vi "Brent Search Powell.vi"(1 "p":dbl[](array[numeric]) format="%.2f", 2 "xit":dbl[](array[numeric]) format="%.2f", 3 "ZEPS":dbl=1e-12 format="%.2e", 6 "Parsed Formula":cluster{"table":i32[][], "result":dbl[]}, 7 "Variables":i32[](array[numeric])=[0, 0], 8 "tol":dbl=1e-06 format="%.2e", 9 "c (start)":dbl=1.0 format="%.2f", 10 "b (start)":dbl=0.5 format="%.2f", 11 "a (start)":dbl format="%.2f") -> (0 "u":dbl=1.5920119327128747e-12 format="%.2f")   [LabVIEW 2024, in "NI_Gmath.lvlib"]
uses:
  NI_Gmath.lvlib
panel:
  in  "fx":dbl=3.25 format="%.2f"
  in  "fw":dbl=2.000000000005184 format="%.2f"
  in  "fv":dbl=2.000000000008388 format="%.2f"
  in  "fu":dbl=2.000000000003184 format="%.2f"
  in  "e":dbl format="%.2f"
  in  "b":dbl format="%.2f"
  in  "a":dbl format="%.2f"
  in  "x":dbl=0.5 format="%.2f"
  in  "w":dbl=2.5920145247273993e-12 format="%.2f"
  in  "v":dbl=4.1939676003423364e-12 format="%.2f"
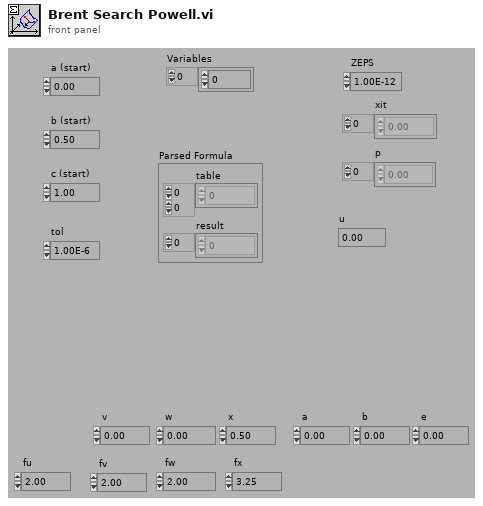
[diagram p1: front panel]
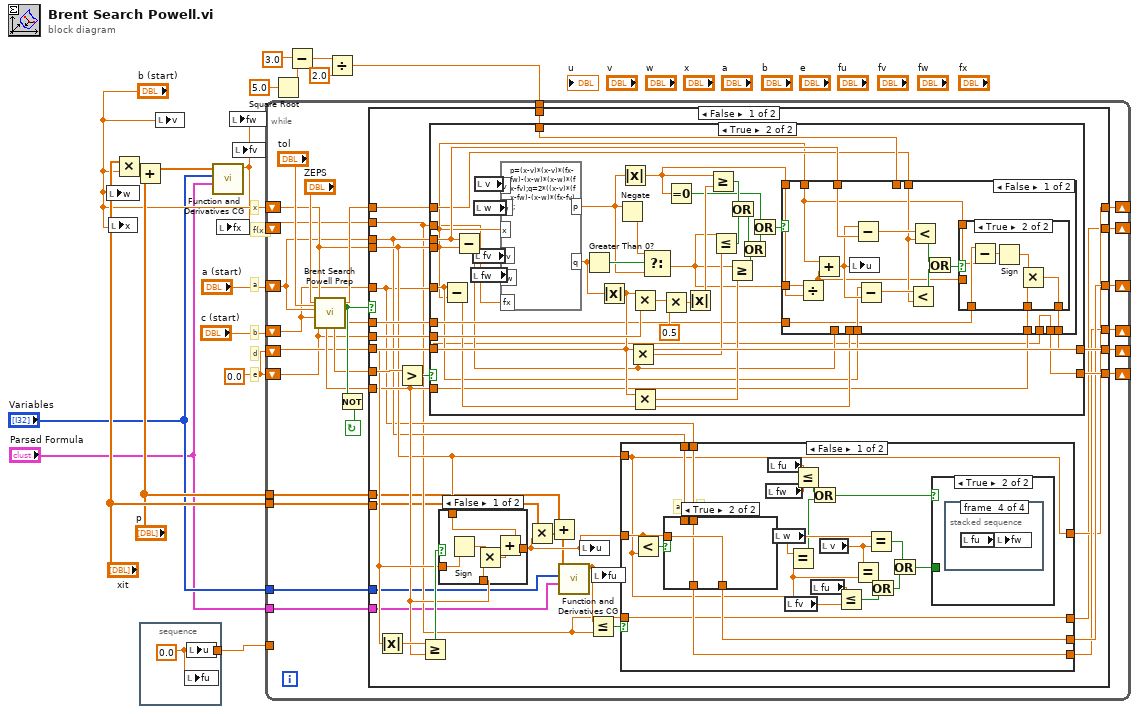
[diagram p0: block diagram]
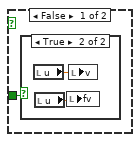
[diagram p2: hidden frame]
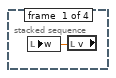
[diagram p4: hidden frame]
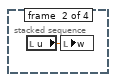
[diagram p5: hidden frame]
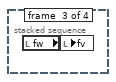
[diagram p6: hidden frame]
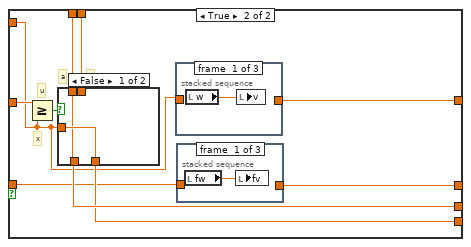
[diagram p8: hidden frame]
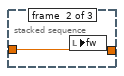
[diagram p9: hidden frame]
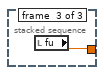
[diagram p10: hidden frame]
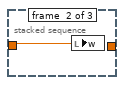
[diagram p11: hidden frame]
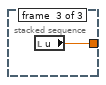
[diagram p12: hidden frame]
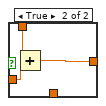
[diagram p14: hidden frame]
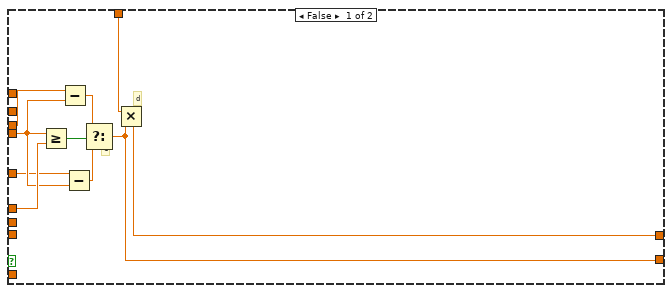
[diagram p15: hidden frame]
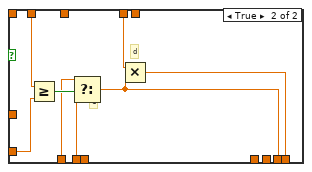
[diagram p17: hidden frame]
diagram:
  w11 = 0.0
  # "d"
  # "e"
  # "f(x)"
  # "x"
  # "b"
  # "a"
  n1 = local write "w"("b (start)") -> ()
  n2 = local write "x"("b (start)") -> ()
  n3 = Multiply(x="xit", y="b (start)") -> (x*y=w10:dbl[])
  n4 = Add(x=w10, y="p") -> (x+y=w9:dbl[])
  n5 = stacked-sequence {
    tunnel: [w19] -> w3
    frame #0 {
      w19 = 0.0
      n6 = local write "fu"(w19) -> ()
      n7 = local write "u"(w19) -> ()
    }
  }
  n8 = local write "v"("b (start)") -> ()
  n9 = call "Function and Derivatives CG.vi"("Parsed Formula"="Parsed Formula", "Variables"="Variables", "X"=w9) -> ("f(X)"=w4:dbl)  [unwired: 7 in, 1 out]
  n10 = local write "fx"(w4) -> ()
  n11 = local write "fw"(w4) -> ()
  n12 = local write "fv"(w4) -> ()
  n13 = Square Root(x=5.0) -> (sqrt(x)=w16:dbl)
  n14 = Subtract(x=3.0, y=w16) -> (x-y=w15:dbl)
  n15 = Divide(x=w15, y=2.0) -> (x/y=w12:dbl)
  n16 = while {
    tunnel: w3 -> [_]
    tunnel: "p" -> [w23]
    tunnel: "xit" -> [w22]
    shift-left: w11 -> [w29]
    shift-right: [w30] -> _
    tunnel: w12 -> [w32]
    shift-left: w11 -> [w28]
    shift-right: [w31] -> _
    shift-left: w4 -> [w36]
    shift-right: [w24] -> _
    shift-left: "b (start)" -> [w41]
    shift-right: [w25] -> _
    shift-left: "c (start)" -> [w33]
    shift-right: [w26] -> _
    shift-left: "a (start)" -> [w34]
    shift-right: [w27] -> _
    tunnel: "Variables" -> [w21]
    tunnel: "Parsed Formula" -> [w20]
    stop <- w39 continue-if-true
    n17 = call "Brent Search Powell Prep.vi"("ZEPS"="ZEPS", "e"=w28, "c (start)"=w33, "tol"="tol", "a (start)"=w34, "b (start)"=w41) -> ("value a"=w35:dbl, "value b"=w38:dbl, "convergence?"=w40:bool, "tol2"=w42:dbl, "value c"=w37:dbl)
    n18 = Not(x=w40) -> (.not. x?=w39:bool)
    n19 = case shown="False" w40 {
      tunnel: w41 -> [w59 _]
      tunnel: w38 -> [w73 w220]
      tunnel: w37 -> [w62 _]
      tunnel: w36 -> [w52 w218]
      tunnel: w35 -> [w71 _]
      tunnel: w34 -> [w58 w217]
      tunnel: w33 -> [w57 w216]
      tunnel: w32 -> [w70 _]
      tunnel: [w69 w220] -> w31
      tunnel: [w63 w221] -> w30
      tunnel: w29 -> [w68 w221]
      tunnel: w28 -> [w67 _]
      tunnel: w42 -> [w66 w219]
      tunnel: [w56 w217] -> w27
      tunnel: [w55 w216] -> w26
      tunnel: [w54 w219] -> w25
      tunnel: [w53 w218] -> w24
      tunnel: w22 -> [w50 _]
      tunnel: w23 -> [w47 _]
      tunnel: w21 -> [w46 _]
      tunnel: w20 -> [w45 _]
      frame False {
        n20 = Greater?(x=w73, y=w62) -> (0:w72:bool)
        n21 = case shown="True" w72 {
          tunnel: w59 -> [w141 w152]
          tunnel: w52 -> [_ w151]
          tunnel: w71 -> [w145 w164]
          tunnel: w58 -> [w140 w157]
          tunnel: w57 -> [w139 w156]
          tunnel: w70 -> [w138 w161]
          tunnel: [w137 w159] -> w69
          tunnel: [w136 w160] -> w63
          tunnel: w68 -> [_ w153]
          tunnel: w67 -> [_ w177]
          tunnel: w66 -> [_ w155]
          tunnel: w62 -> [_ w154]
          frame False {
            # "d"
            # "e"
            n22 = Greater Or Equal?(x=w141, y=w145) -> (x >= y?=w144:bool)
            n23 = Subtract(x=w140, y=w141) -> (x-y=w142:dbl)
            n24 = Subtract(x=w139, y=w141) -> (x-y=w143:dbl)
            n25 = Select(t=w142, s=w144, f=w143) -> (s? t:f=w137:dbl)
            n26 = Multiply(x=w138, y=w137) -> (x*y=w136:dbl)
          }
          frame True {
            n27 = Subtract(x=w156, y=w152) -> (x-y=w162:dbl)
            n28 = Subtract(x=w157, y=w152) -> (x-y=w163:dbl)
            n29 = local read "fw"() -> (w180:dbl)
            n30 = local read "fv"() -> (w181:dbl)
            n31 = local read "w"() -> (w182:dbl)
            n32 = local read "v"() -> (w183:dbl)
            n33 = formula code="p=(x-v)*(x-v)*(fx-fw)-(x-w)*(x-w)*(fx-fv);q=2*((x-v)*(fx-fw)-(x-w)*(fx-fv));"("v"=w183, "w"=w182, "x"=w152, "fv"=w181, "fw"=w180, "fx"=w151) -> ("p"=w147:dbl, "q"=w172:dbl)
            n34 = Greater Than 0?(x=w172) -> (x > 0?=w179:bool)
            n35 = Absolute Value(x=w172) -> (abs(x)=w171:dbl)
            n36 = Negate(x=w147) -> (-x=w178:dbl)
            n37 = Absolute Value(x=w147) -> (abs(x)=w146:dbl)
            n38 = Multiply(x=w171, y=w163) -> (x*y=w170:dbl)
            n39 = Multiply(x=w171, y=w177) -> (x*y=w176:dbl)
            n40 = Multiply(x=w171, y=w162) -> (x*y=w169:dbl)
            n41 = Select(t=w178, s=w179, f=w147) -> (s? t:f=w158:dbl)
            n42 = Multiply(x=w176, y=0.5) -> (x*y=w174:dbl)
            n43 = Equal To 0?(x=w146) -> (x = 0?=w149:bool)
            n44 = Absolute Value(x=w174) -> (abs(x)=w173:dbl)
            n45 = Greater Or Equal?(x=w146, y=w173) -> (x >= y?=w168:bool)
            n46 = Less Or Equal?(x=w158, y=w170) -> (x <= y?=w167:bool)
            n47 = Greater Or Equal?(x=w158, y=w169) -> (x >= y?=w165:bool)
            n48 = Or(x=w168, y=w167) -> (x .or. y?=w166:bool)
            n49 = Or(x=w166, y=w165) -> (x .or. y?=w150:bool)
            n50 = Or(x=w149, y=w150) -> (x .or. y?=w148:bool)
            n51 = case shown="False" w148 {
              tunnel: w152 -> [w187 w214]
              tunnel: w164 -> [w188 w213]
              tunnel: w163 -> [_ w212]
              tunnel: w162 -> [_ w211]
              tunnel: w161 -> [_ w210]
              tunnel: [w185 w209] -> w160
              tunnel: [w184 w208] -> w159
              tunnel: w158 -> [w200 _]
              tunnel: w146 -> [w199 _]
              tunnel: w157 -> [w198 _]
              tunnel: w156 -> [w196 _]
              tunnel: w155 -> [w193 _]
              tunnel: w154 -> [w186 _]
              tunnel: w153 -> [w184 _]
              frame False {
                n52 = Divide(x=w200, y=w199) -> (x/y=w189:dbl)
                n53 = Add(x=w187, y=w189) -> (x+y=w197:dbl)
                n54 = local write "u"(w197) -> ()
                n55 = Subtract(x=w197, y=w198) -> (x-y=w195:dbl)
                n56 = Subtract(x=w196, y=w197) -> (x-y=w194:dbl)
                n57 = Less?(x=w194, y=w193) -> (x < y?=w191:bool)
                n58 = Less?(x=w195, y=w193) -> (x < y?=w192:bool)
                n59 = Or(x=w192, y=w191) -> (x .or. y?=w190:bool)
                n60 = case shown="True" w190 {
                  tunnel: w189 -> [w201 _]
                  tunnel: w188 -> [_ w207]
                  tunnel: w187 -> [_ w206]
                  tunnel: w186 -> [_ w203]
                  tunnel: [w201 w202] -> w185
                  frame False {
                  }
                  frame True {
                    n61 = Subtract(x=w207, y=w206) -> (x-y=w205:dbl)
                    n62 = Sign(1:w205) -> (0:w204:dbl)
                    n63 = Multiply(x=w204, y=w203) -> (x*y=w202:dbl)
                  }
                }
              }
              frame True {
                # "d"
                # "e"
                n64 = Greater Or Equal?(x=w214, y=w213) -> (x >= y?=w215:bool)
                n65 = Select(t=w212, s=w215, f=w211) -> (s? t:f=w208:dbl)
                n66 = Multiply(x=w210, y=w208) -> (x*y=w209:dbl)
              }
            }
          }
        }
        n67 = Absolute Value(x=w63) -> (abs(x)=w64:dbl)
        n68 = Greater Or Equal?(x=w64, y=w62) -> (x >= y?=w65:bool)
        n69 = case shown="False" w65 {
          tunnel: w63 -> [w132 w135]
          tunnel: w59 -> [w128 w134]
          tunnel: w62 -> [w130 _]
          tunnel: [w127 w133] -> w51
          frame False {
            n70 = Sign(1:w132) -> (0:w131:dbl)
            n71 = Multiply(x=w131, y=w130) -> (x*y=w129:dbl)
            n72 = Add(x=w128, y=w129) -> (x+y=w127:dbl)
          }
          frame True {
            n73 = Add(x=w134, y=w135) -> (x+y=w133:dbl)
          }
        }
        n74 = Multiply(x=w50, y=w51) -> (x*y=w49:dbl[])
        n75 = Add(x=w47, y=w49) -> (x+y=w48:dbl[])
        n76 = call "Function and Derivatives CG.vi"("Parsed Formula"=w45, "Variables"=w46, "X"=w48) -> ("f(X)"=w61:dbl)  [unwired: 7 in, 1 out]
        n77 = local write "u"(w51) -> ()
        n78 = Less Or Equal?(x=w61, y=w52) -> (x <= y?=w60:bool)
        n79 = local write "fu"(w61) -> ()
        n80 = case shown="False" w60 {
          tunnel: w51 -> [w92 w116]
          tunnel: w59 -> [w75 w110]
          tunnel: w58 -> [w94 w114]
          tunnel: w57 -> [w93 w113]
          tunnel: [w90 w112] -> w56
          tunnel: [w91 w111] -> w55
          tunnel: [w75 w109] -> w54
          tunnel: [w74 w108] -> w53
          tunnel: w52 -> [w74 w107]
          frame False {
            # "b"
            # "a"
            n81 = Less?(x=w92, y=w75) -> (x < y?=w95:bool)
            n82 = case shown="True" w95 {
              tunnel: w94 -> [w104 _]
              tunnel: w93 -> [_ w105]
              tunnel: [w104 w106] -> w90
              tunnel: w92 -> [w103 w106]
              tunnel: [w103 w105] -> w91
              frame False {
              }
              frame True {
              }
            }
            n83 = local read "fw"() -> (w88:dbl)
            n84 = local read "fu"() -> (w89:dbl)
            n85 = local read "w"() -> (w87:dbl)
            n86 = local read "fv"() -> (w83:dbl)
            n87 = Equal?(x=w87, y=w75) -> (x = y?=w86:bool)
            n88 = Less Or Equal?(x=w89, y=w88) -> (x <= y?=w85:bool)
            n89 = Or(x=w85, y=w86) -> (x .or. y?=w84:bool)
            n90 = local read "fu"() -> (w82:dbl)
            n91 = local read "v"() -> (w79:dbl)
            n92 = Less Or Equal?(x=w82, y=w83) -> (x <= y?=w80:bool)
            n93 = Equal?(x=w79, y=w75) -> (x = y?=w81:bool)
            n94 = Equal?(x=w87, y=w79) -> (x = y?=w78:bool)
            n95 = Or(x=w81, y=w80) -> (x .or. y?=w77:bool)
            n96 = Or(x=w78, y=w77) -> (x .or. y?=w76:bool)
            n97 = case shown="True" w84 {
              tunnel: w76 -> [w96 _]
              frame False {
                n98 = case shown="True" w96 {
                  frame False {
                  }
                  frame True {
                    n99 = local read "u"() -> (w98:dbl)
                    n100 = local read "u"() -> (w97:dbl)
                    n101 = local write "fv"(w97) -> ()
                    n102 = local write "v"(w98) -> ()
                  }
                }
              }
              frame True {
                n103 = stacked-sequence {
                  frame #0 {
                    n104 = local read "v"() -> (w99:dbl)
                    n105 = local write "w"(w99) -> ()
                  }
                  frame #1 {
                    n106 = local read "u"() -> (w100:dbl)
                    n107 = local write "w"(w100) -> ()
                  }
                  frame #2 {
                    n108 = local read "fw"() -> (w101:dbl)
                    n109 = local write "fv"(w101) -> ()
                  }
                  frame #3 {
                    n110 = local read "fu"() -> (w102:dbl)
                    n111 = local write "fw"(w102) -> ()
                  }
                }
              }
            }
          }
          frame True {
            # "b"
            # "a"
            # "u"
            # "x"
            n112 = Greater Or Equal?(x=w116, y=w110) -> (x >= y?=w115:bool)
            n113 = case shown="False" w115 {
              tunnel: w114 -> [w123 _]
              tunnel: w113 -> [_ w125]
              tunnel: [w123 w126] -> w112
              tunnel: w110 -> [w124 w126]
              tunnel: [w124 w125] -> w111
              frame False {
              }
              frame True {
              }
            }
            n114 = stacked-sequence {
              tunnel: w110 -> [_ w121 _]
              tunnel: [_ _ w122] -> w109
              frame #0 {
                n115 = local read "w"() -> (w120:dbl)
                n116 = local write "v"(w120) -> ()
              }
              frame #1 {
                n117 = local write "w"(w121) -> ()
              }
              frame #2 {
                n118 = local read "u"() -> (w122:dbl)
              }
            }
            n119 = stacked-sequence {
              tunnel: w107 -> [_ w118 _]
              tunnel: [_ _ w119] -> w108
              frame #0 {
                n120 = local read "fw"() -> (w117:dbl)
                n121 = local write "fv"(w117) -> ()
              }
              frame #1 {
                n122 = local write "fw"(w118) -> ()
              }
              frame #2 {
                n123 = local read "fu"() -> (w119:dbl)
              }
            }
          }
        }
      }
      frame True {
      }
    }
  }
